vi "Create From Variant (String).vi"(8 "error in (no error)":errorcluster, 10 "Variant":variant, 11 "JSON String in":refnum<class "JSON Value.lvclass">) -> (0 "error out":errorcluster, 3 "JSON String out":refnum<class "JSON Value.lvclass">)   [LabVIEW 2016, in "JSFL Variant Support.lvlib"]
doc: "Creates a new JSON instance from the given Variant."
uses:
  JSFL Variant Support.lvlib
  JSON Value.lvclass
  JSON Value.lvclass/JSON Value.ctl
  subVIs/Write value.vi
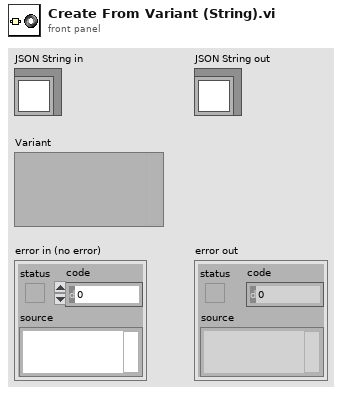
[diagram p1: front panel]
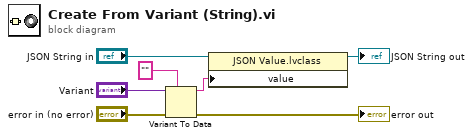
[diagram p0: block diagram]
diagram:
  n1 = Variant To Data(error in="error in (no error)", type="", Variant="Variant") -> (data=w2:string, error out=→"error out":errorcluster)
  n2 = property class="JSON Value.lvclass"(reference="JSON String in", "value"=w2) -> (reference out=→"JSON String out":refnum<class "JSON Value.lvclass">)  [unwired: 1 in, 1 out]
